vi "SUB-BLE Rx data-CDC IMU.vi"(8 "data in":u8[](array[numeric]) format="%2x") -> (0 "IMU data":T1 caption="IMU Monitoring data" {"Accelerometer Z" format="%#.9f"; "Accelerometer Y" format="%#.9f"; "Accelerometer X" format="%#.9f"; "Gyroscope Z" format="%#.9f"; "Gyroscope Y" format="%#.9f"; "Gyroscope X" format="%#.9f"}, 1 "CDC data":T2 caption="CDC Monitoring data" {"Right Wing-C, C6/C0" format="%#.9f"; "Right Wing-B, C5/C0" format="%#.9f"; "Right Wing-A, C4/C0" format="%#.9f"; "Left Wing-C, C3/C0" format="%#.9f"; "Left Wing-B, C2/C0" format="%#.9f"; "Left Wing-A, C1/C0" format="%#.9f"}, 2 "Bat":u16, 3 "*Board ID":string="None...." caption="S/N")   [LabVIEW 2015]
doc: "Use this template to create an application that executes repeatedly until you click the Stop button. This template polls the state of the Stop button and does not use events. Use the Top-Level Application template (not available in the Base package) to create a single-loop application with event handling."
panel:
  out "BLE Packet (buf)":u8[](array[numeric])
  out "BLE Packet (data)":u8[](array[numeric])
  # "BLE 수신 데이터를 분류: Monitoring/Setting data"
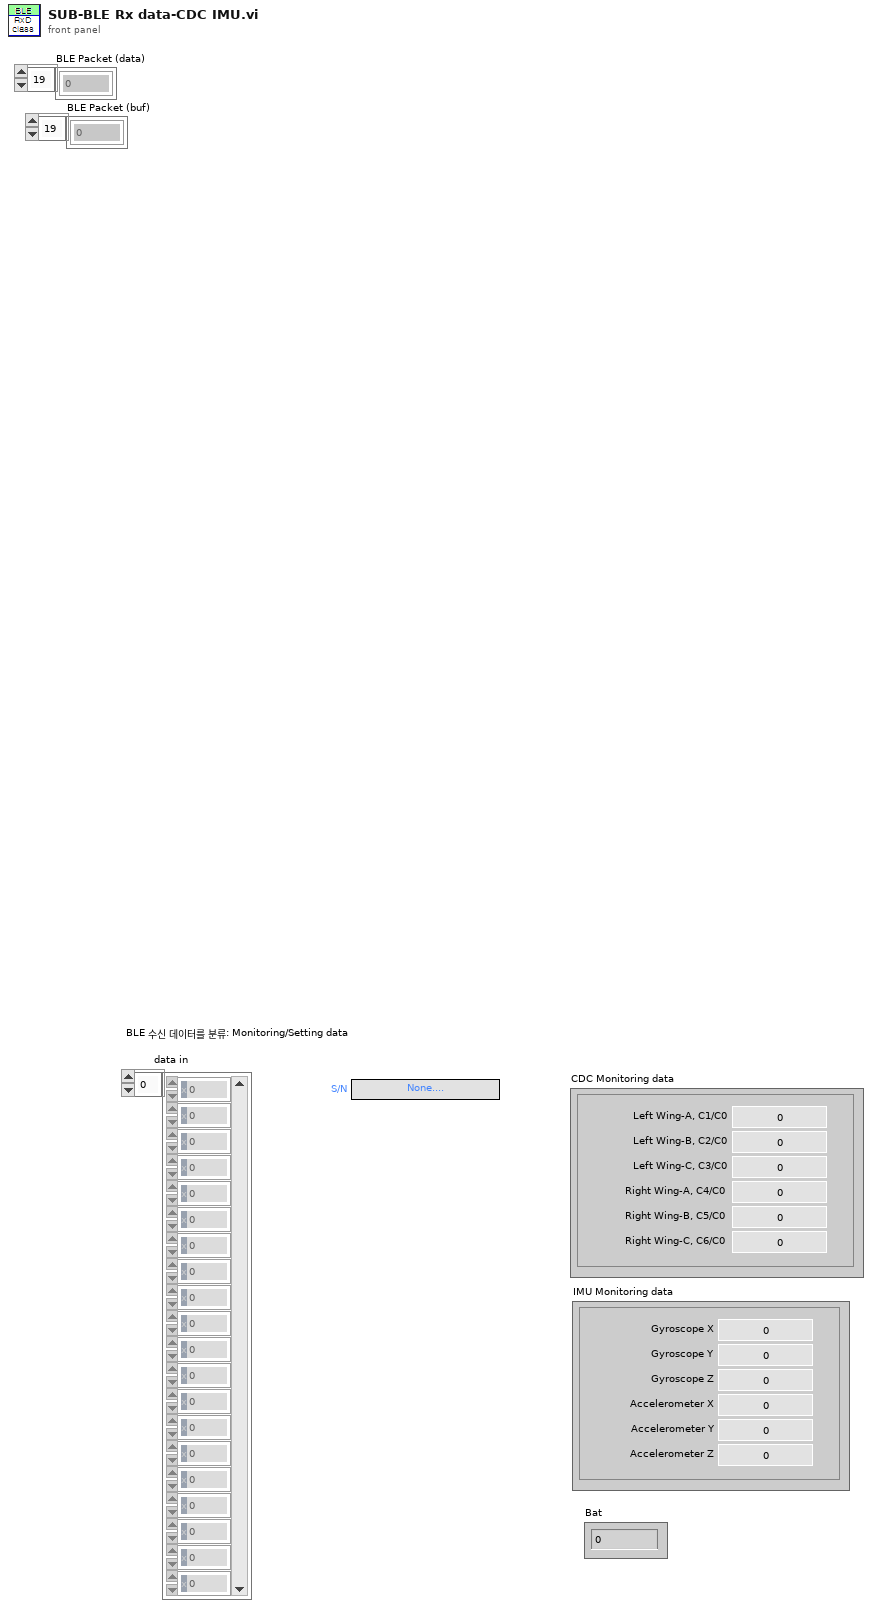
[diagram p1: front panel]
types:
  T1 = typedef "컨트롤-IMU data.ctl" = cluster{"Gyroscope X":dbl, "Gyroscope Y":dbl, "Gyroscope Z":dbl, "Accelerometer X":dbl, "Accelerometer Y":dbl, "Accelerometer Z":dbl}
  T2 = typedef "컨트롤-CDC data.ctl" = cluster{"Left Wing-A, C1/C0":dbl, "Left Wing-B, C2/C0":dbl, "Left Wing-C, C3/C0":dbl, "Right Wing-A, C4/C0":dbl, "Right Wing-B, C5/C0":dbl, "Right Wing-C, C6/C0":dbl}
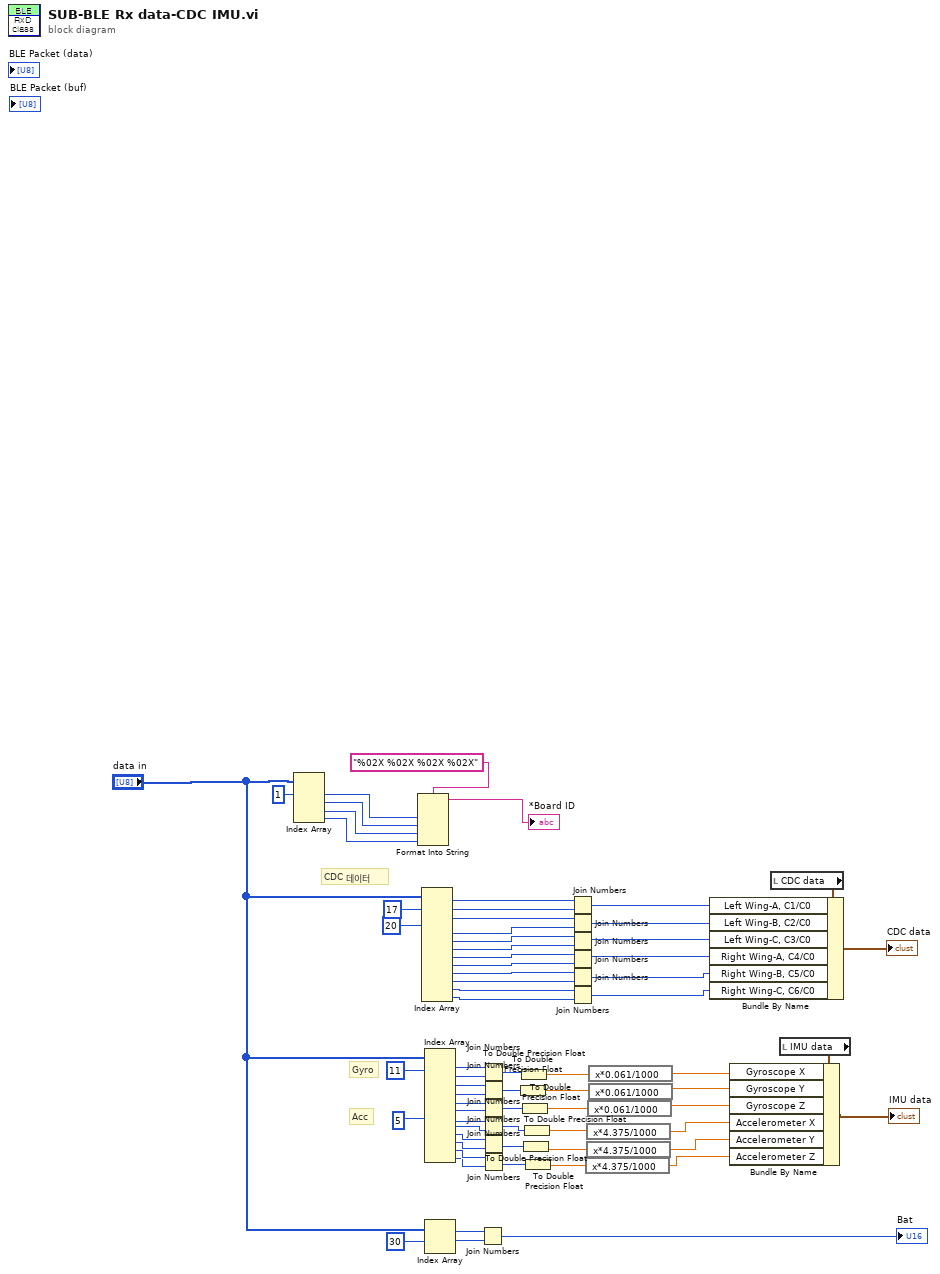
[diagram p0: block diagram]
diagram:
  # "Acc"
  # "Gyro"
  # "CDC 데이터"
  n1 = Index Array(array="data in", index #1=1 ("인덱스")) -> (element #1=w66:u8, element #2=w65:u8, element #3=w64:u8, element #4=w63:u8)  [unwired: 3 in]
  n2 = Format Into String(format string="%02X %02X %02X %02X" ("구분 문자(탭)"), w66, w65, w64, w63) -> (resulting string=→"*Board ID":string)  [unwired: 2 in, 1 out]
  n3 = Index Array(array="data in", index #1=17 ("인덱스"), index #3=20 ("인덱스")) -> (element #1=w59:u8, element #2=w58:u8, element #3=w57:u8, element #4=w56:u8, element #5=w55:u8, element #6=w54:u8, element #7=w53:u8, element #8=w52:u8, element #9=w51:u8, element #10=w50:u8, element #11=w49:u8, element #12=w48:u8)  [unwired: 10 in]
  n4 = Index Array(array="data in", index #1=11 ("인덱스"), index #7=5 ("인덱스")) -> (element #1=w37:u8, element #2=w36:u8, element #3=w35:u8, element #4=w34:u8, element #5=w33:u8, element #6=w32:u8, element #7=w31:u8, element #8=w30:u8, element #9=w29:u8, element #10=w28:u8, element #11=w27:u8, element #12=w26:u8)  [unwired: 10 in]
  n5 = Index Array(array="data in", index #1=30 ("인덱스")) -> (element #1=w4:u8, element #2=w5:u8)  [unwired: 1 in]
  n6 = Join Numbers(hi=w4, lo=w5) -> ((hi.lo)=→"Bat":u16)
  n7 = Join Numbers(hi=w37, lo=w36) -> ((hi.lo)=w24:u16)
  n8 = Join Numbers(hi=w35, lo=w34) -> ((hi.lo)=w19:u16)
  n9 = Join Numbers(hi=w33, lo=w32) -> ((hi.lo)=w20:u16)
  n10 = Join Numbers(hi=w31, lo=w30) -> ((hi.lo)=w23:u16)
  n11 = Join Numbers(hi=w29, lo=w28) -> ((hi.lo)=w22:u16)
  n12 = Join Numbers(hi=w27, lo=w26) -> ((hi.lo)=w21:u16)
  n13 = To Double Precision Float(number=w19) -> (double precision float=w13:dbl)
  n14 = To Double Precision Float(number=w24) -> (double precision float=w18:dbl)
  n15 = To Double Precision Float(number=w20) -> (double precision float=w14:dbl)
  n16 = To Double Precision Float(number=w22) -> (double precision float=w16:dbl)
  n17 = To Double Precision Float(number=w23) -> (double precision float=w17:dbl)
  n18 = To Double Precision Float(number=w21) -> (double precision float=w15:dbl)
  n19 = Join Numbers(hi=w59, lo=w58) -> ((hi.lo)=w45:u16)
  n20 = Join Numbers(hi=w57, lo=w56) -> ((hi.lo)=w44:u16)
  n21 = Join Numbers(hi=w55, lo=w54) -> ((hi.lo)=w43:u16)
  n22 = Join Numbers(hi=w53, lo=w52) -> ((hi.lo)=w42:u16)
  n23 = Join Numbers(hi=w51, lo=w50) -> ((hi.lo)=w41:u16)
  n24 = Join Numbers(hi=w49, lo=w48) -> ((hi.lo)=w40:u16)
  n25 = expression code="x*4.375/1000"(w15) -> (w6:dbl)
  n26 = expression code="x*4.375/1000"(w17) -> (w8:dbl)
  n27 = expression code="x*4.375/1000"(w16) -> (w7:dbl)
  n28 = expression code="x*0.061/1000"(w14) -> (w9:dbl)
  n29 = expression code="x*0.061/1000"(w18) -> (w11:dbl)
  n30 = expression code="x*0.061/1000"(w13) -> (w10:dbl)
  n31 = local read "CDC data"() -> (w61:T2)
  n32 = Bundle By Name(cluster=w61, "Left Wing-A, C1/C0"=w45, "Left Wing-B, C2/C0"=w44, "Left Wing-C, C3/C0"=w43, "Right Wing-A, C4/C0"=w42, "Right Wing-B, C5/C0"=w41, "Right Wing-C, C6/C0"=w40) -> (→"CDC data":T2)
  n33 = local read "IMU data"() -> (w39:T1)
  n34 = Bundle By Name(cluster=w39, "Gyroscope X"=w11, "Gyroscope Y"=w10, "Gyroscope Z"=w9, "Accelerometer X"=w8, "Accelerometer Y"=w7, "Accelerometer Z"=w6) -> (→"IMU data":T1)
